vi "Write Pressure Servo Valve 1 Setpoint.vi"(10 "Pressure Servo Valve 1 Setpoint":dbl[unit], 11 "IActuatorCylinder in":refnum<class "IActuatorCylinder.lvclass">) -> (3 "IActuatorCylinder out":refnum<class "IActuatorCylinder.lvclass">)   [LabVIEW 2015, in "IActuatorCylinder.lvclass"]
uses:
  IActuatorCylinder.lvclass
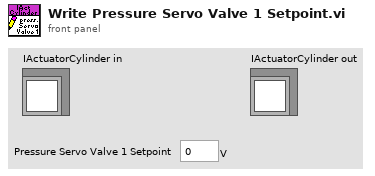
[diagram p1: front panel]
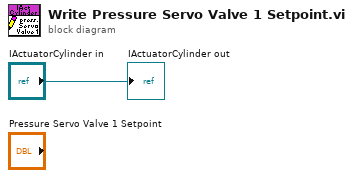
[diagram p0: block diagram]
diagram:
  "IActuatorCylinder out" <- "IActuatorCylinder in"
